vi "ManageScript.vi"(6 "Severity":string="Critical", 7 "ErrorIn Array":errorcluster[](array[cluster]), 10 "Script Locations":path[](array[path])) -> (0 "ErrorOut Array":errorcluster[](array[cluster]))   [LabVIEW 2018, in "Test.lvclass"]
uses:
  Test.lvclass
  <vilib>/Utility/config.llb/NI_LVConfig.lvlib
  <userlib>/NIST/NISTErrorLib/NISTErrorLib.lvlib
panel:
  in  "Script to Edit":string[](array[string])
  out "Script to View":string
  in  "btnRead":bool
  out "Numeric Control":i32
  out "Array 4":bool[](array[boolean])
  in  "Save As":bool
  in  "Save Button":bool
  in  "Script Names":string[](array[string])
  in  "Close Button":bool
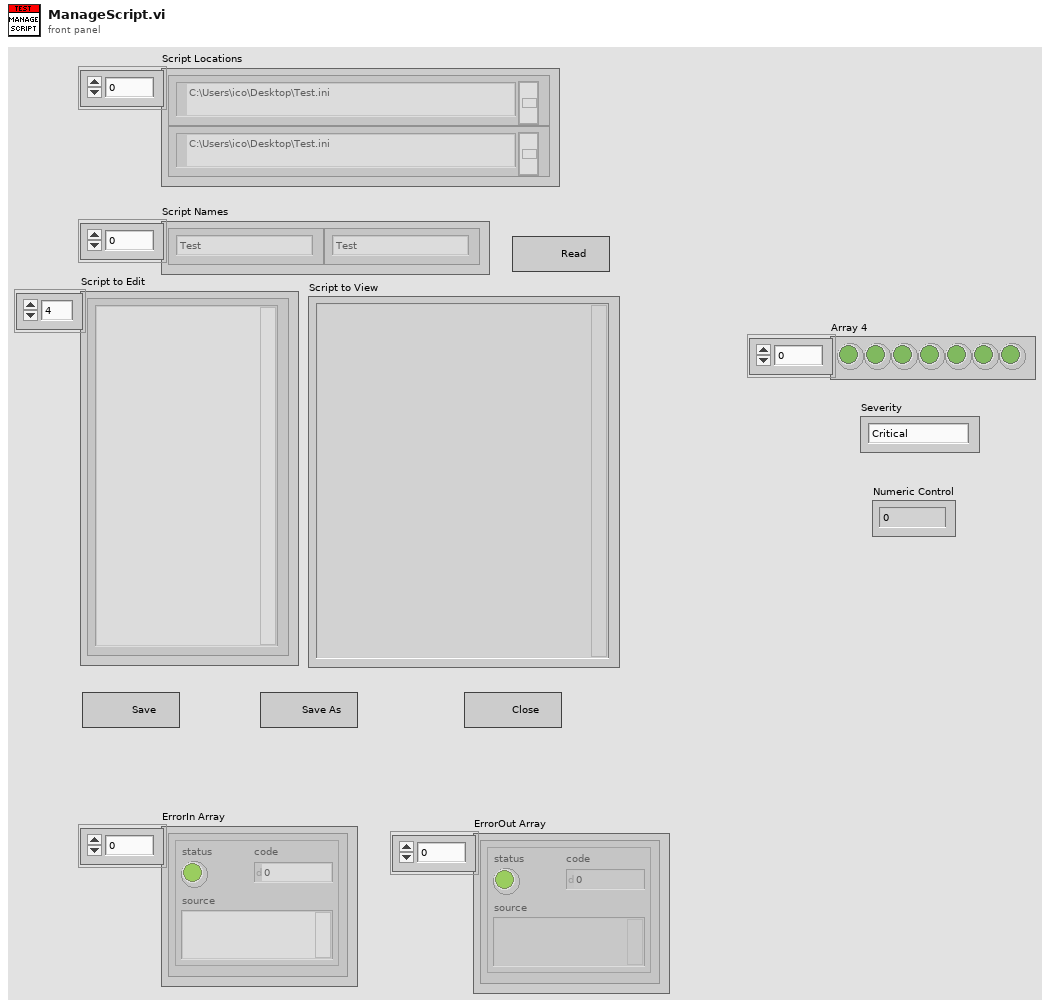
[diagram p1: front panel]
types:
  T1 = enum32{"Invalid", "Standard", "Closed", "Hidden", "Minimized", "Maximized"}
  T2 = enum32{"Invalid", "Default", "Floating", "Floating/Auto-Hide", "Modal"}
  T3 = typedef "NI_LVConfig.lvlib/Config Data RefNum.ctl" = refnum<k1>
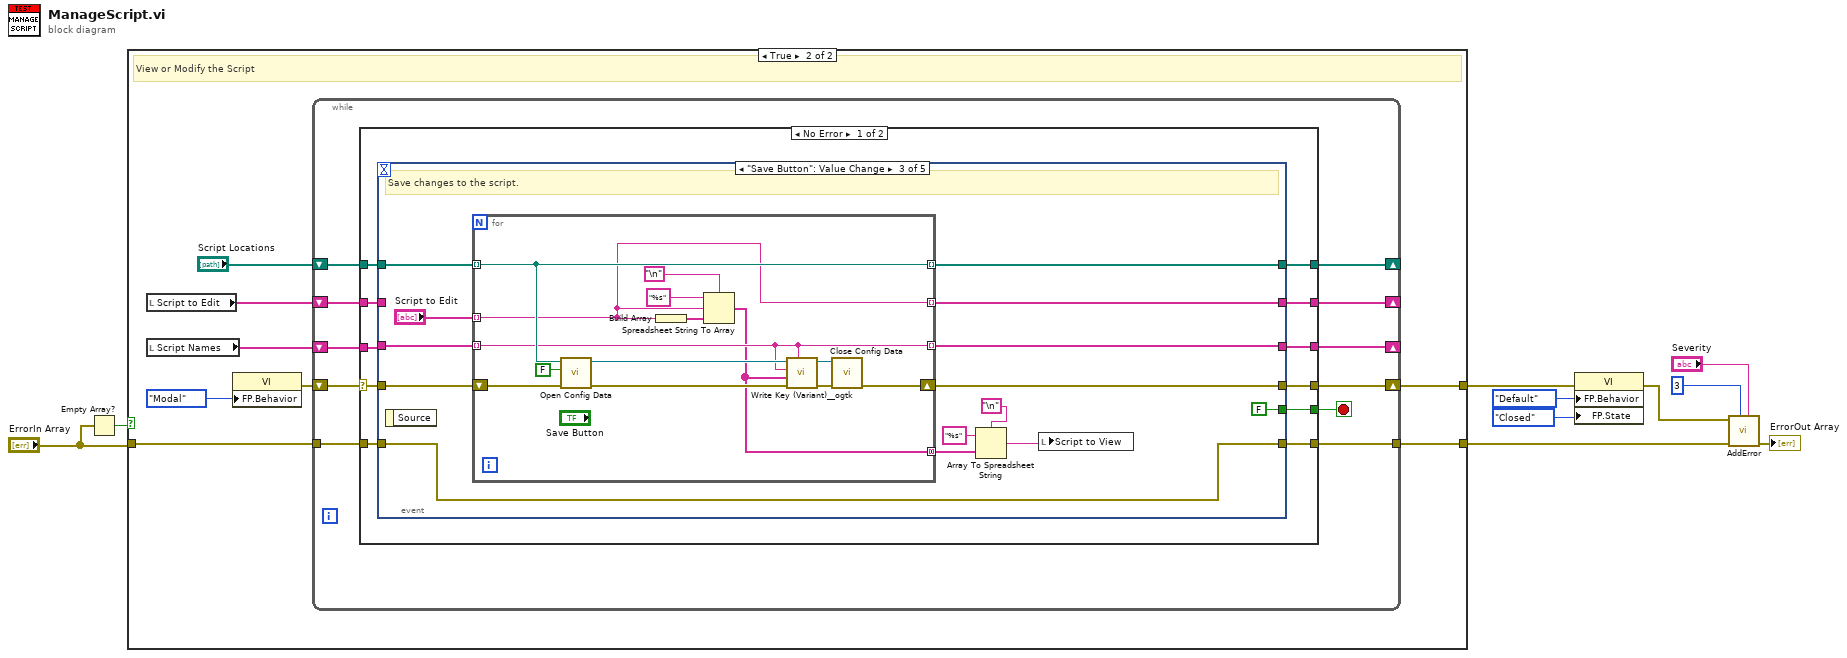
[diagram p0: block diagram]
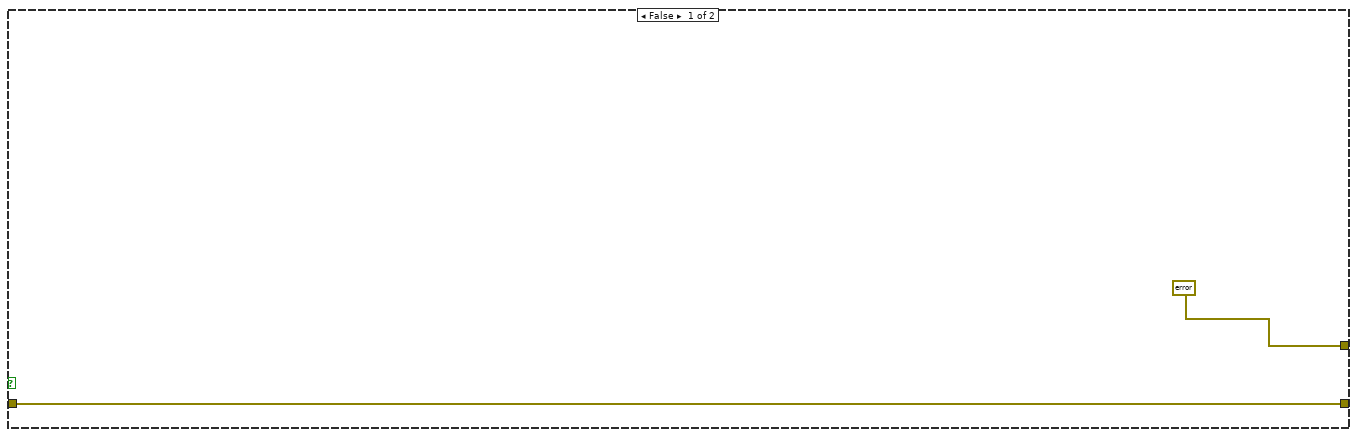
[diagram p2: hidden frame]
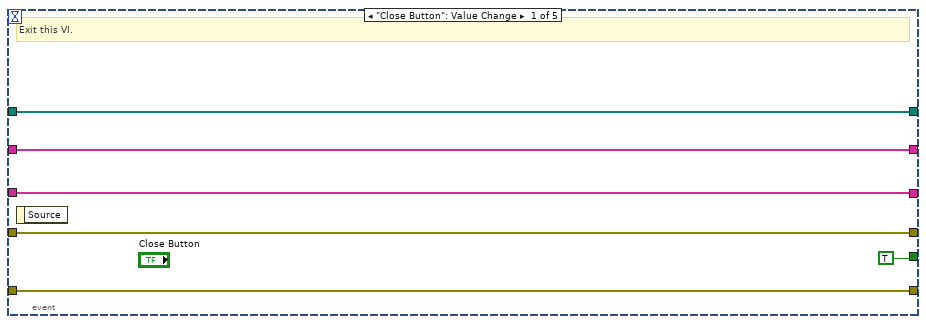
[diagram p3: hidden frame]
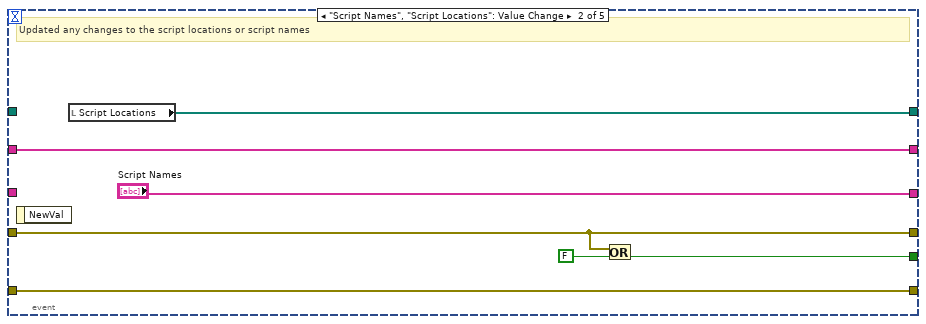
[diagram p4: hidden frame]
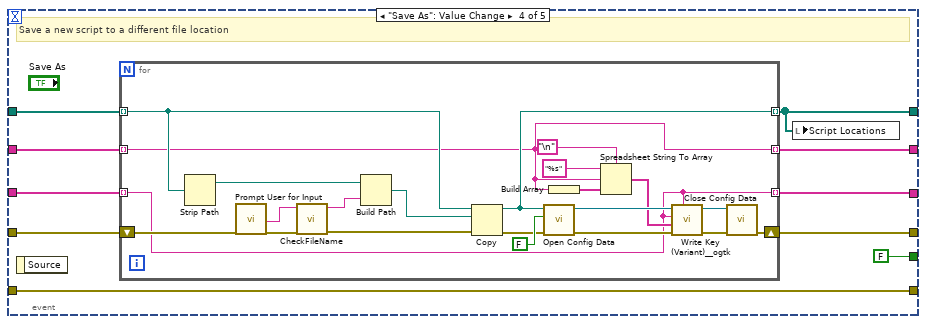
[diagram p5: hidden frame]
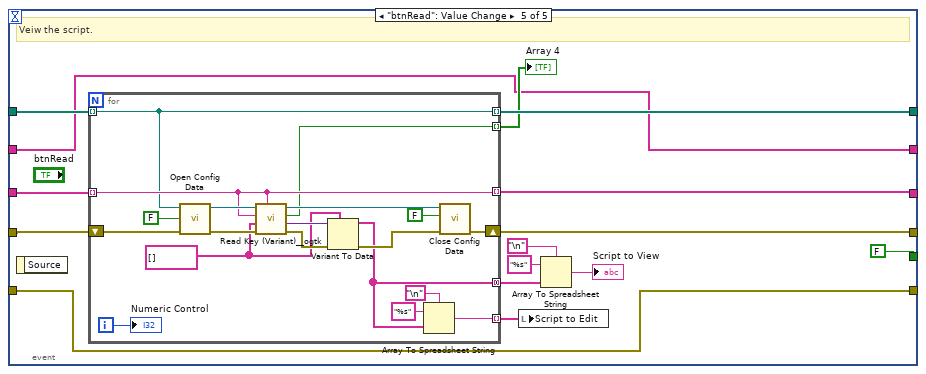
[diagram p6: hidden frame]
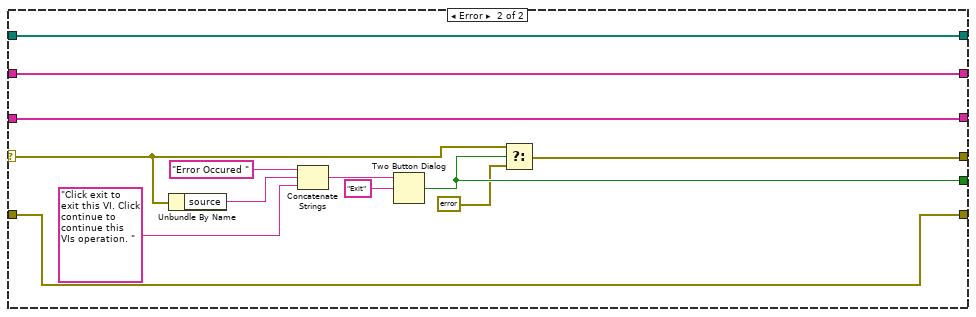
[diagram p7: hidden frame]
diagram:
  n1 = Empty Array?(array="ErrorIn Array") -> (empty?=w10:bool)
  n2 = case shown="True" w10 {
    tunnel: "ErrorIn Array" -> [w12 w20]
    tunnel: [w12 w14] -> w1
    tunnel: [errorcluster {"status"=FALSE, "code"=0, "source"=""} ("error out") w15] -> w3
    frame False {
    }
    frame True {
      # "View or Modify the Script"
      n3 = local read "Script to Edit"() -> (w16:string[])
      n4 = local read "Script Names"() -> (w17:string[])
      n5 = property class="VI"("FP.Behavior"=T2."Modal" ("Front Panel Window:Behavior")) -> (error out=w19:errorcluster)  [unwired: 2 in, 1 out]
      n6 = while {
        tunnel: w20 -> [w30]
        tunnel: [w29] -> w14
        shift-right: [w27] -> w15
        shift-left: w19 -> [w28]
        shift-right: [w25] -> _
        shift-left: "Script Locations" -> [w26]
        shift-right: [w23] -> _
        shift-left: w17 -> [w24]
        shift-right: [w21] -> _
        shift-left: w16 -> [w22]
        stop <- w31 stop-if-true
        n7 = case shown="No Error" w28 {
          selector: w28 -> [w39 w152]
          tunnel: [w42 w151] -> w31
          tunnel: w30 -> [w41 w156]
          tunnel: [w40 w156] -> w29
          tunnel: [w38 w153] -> w27
          tunnel: w26 -> [w37 w162]
          tunnel: [w36 w162] -> w25
          tunnel: w24 -> [w35 w160]
          tunnel: [w34 w160] -> w23
          tunnel: w22 -> [w33 w161]
          tunnel: [w32 w161] -> w21
          frame No Error {
            n8 = event shown="[2] \"Save Button\": Value Change" {
              selector: _ -> [_ _ _ _ _]
              dyn-events: _ -> [_ _ _ _ _]
              timeout: _ -> [_ _ _ _ _]
              tunnel: [TRUE w52 FALSE FALSE FALSE] -> w42
              tunnel: w41 -> [w48 w54 w60 w92 w126]
              tunnel: [w48 w54 w60 w92 w126] -> w40
              tunnel: w37 -> [w45 _ w68 w91 w128]
              tunnel: w35 -> [w44 _ w66 w90 w127]
              tunnel: w39 -> [w46 w51 w69 w93 w130]
              tunnel: [w46 w51 w64 w89 w129] -> w38
              tunnel: [w45 w49 w65 w84 w120] -> w36
              tunnel: [w44 "Script Names" w62 w87 w125] -> w34
              tunnel: w33 -> [w43 w50 _ w86 w117]
              tunnel: [w43 w50 w61 w85 w117] -> w32
              event "Close Button": Value Change {
                # "Exit this VI."
                n9 = event-data() -> ()  [unwired: 1 in, 1 out]
              }
              event "Script Names", "Script Locations": Value Change {
                # "Updated any changes to the script locations or script names"
                n10 = event-data() -> ()  [unwired: 1 in, 1 out]
                n11 = local read "Script Locations"() -> (w49:path[])
                n12 = Or(x=w51, y=FALSE) -> (x .or. y?=w52:bool)
              }
              event "Save Button": Value Change {
                # "Save changes to the script."
                n13 = event-data() -> ()  [unwired: 1 in, 1 out]
                n14 = for {
                  shift-right: [w77] -> w64
                  shift-left: w69 -> [w78]
                  tunnel: w68 -> [w73] mode=indexing
                  tunnel: "Script to Edit" -> [w71] mode=indexing
                  tunnel: w66 -> [w72] mode=indexing
                  tunnel: [w73] -> w65 mode=indexing
                  tunnel: [w72] -> w62 mode=indexing
                  tunnel: [w71] -> w61 mode=indexing
                  tunnel: [w70] -> w59 mode=concatenating
                  n15 = call <vilib>:"Open Config Data.vi"("error in (no error)"=w78, "create file if necessary (T)"=FALSE, "configuration file path"=w73) -> ("error out"=w82:errorcluster, "refnum"=w80:T3)  [unwired: 6 in, 1 out]
                  n16 = Build Array(w71) -> (w76:string[])
                  n17 = Spreadsheet String To Array(delimiter (Tab)="\n", format string="%s", spreadsheet string=w71, array type (2D Dbl)=w76) -> (array=w70:string[])
                  n18 = call <userlib>:"Write Key (Variant)__ogtk.vi"("section"=w72, "error in (no error)"=w82, "key-value"=w70, "key (optional)"=w72, "refnum"=w80) -> ("error out"=w81:errorcluster, "refnum out"=w79:T3)  [unwired: 5 in]
                  n19 = call <vilib>:"Close Config Data.vi"("error in (no error)"=w81, "refnum"=w79) -> ("error out"=w77:errorcluster)  [unwired: 8 in, 1 out]
                }
                n20 = Array To Spreadsheet String(delimiter (Tab)="\n", array=w59, 3:"%s" ("format string")) -> (spreadsheet string=w56:string)
                n21 = local write "Script to View"(w56) -> ()
              }
              event "Save As": Value Change {
                # "Save a new script to a different file location"
                n22 = event-data() -> ()  [unwired: 1 in, 1 out]
                n23 = for {
                  shift-right: [w110] -> w89
                  shift-left: w93 -> [w102]
                  tunnel: w91 -> [w101] mode=indexing
                  tunnel: w86 -> [w98] mode=indexing
                  tunnel: w90 -> [w99] mode=indexing
                  tunnel: [w100] -> w84 mode=indexing
                  tunnel: [w99] -> w87 mode=indexing
                  tunnel: [w98] -> w85 mode=indexing
                  n24 = Strip Path(path=w101) -> (stripped path=w104:path)  [unwired: 1 out]
                  n25 = call "Prompt User for Input"("error in (no error)"=w102) -> ("File Name"=w96:string, "error out"=w97:errorcluster)  [unwired: 16 in, 1 out]
                  n26 = call "CheckFileName.vi"("Error In"=w97, "File Name in"=w96) -> ("Error Out"=w94:errorcluster, "File Name out"=w95:string)  [unwired: 8 in]
                  n27 = Build Path(base path=w104, name or relative path=w95) -> (appended path=w105:path)
                  n28 = Copy(8:w94, 10:w105, 11:w101) -> (0:w103:errorcluster, 3:w100:path)  [unwired: 2 in, 1 out]
                  n29 = call <vilib>:"Open Config Data.vi"("error in (no error)"=w103, "create file if necessary (T)"=FALSE, "configuration file path"=w100) -> ("error out"=w114:errorcluster, "refnum"=w112:T3)  [unwired: 6 in, 1 out]
                  n30 = Build Array(w98) -> (w109:string[])
                  n31 = Spreadsheet String To Array(delimiter (Tab)="\n", format string="%s", spreadsheet string=w98, array type (2D Dbl)=w109) -> (array=w106:string[])
                  n32 = call <userlib>:"Write Key (Variant)__ogtk.vi"("section"=w99, "error in (no error)"=w114, "key-value"=w106, "key (optional)"=w99, "refnum"=w112) -> ("error out"=w113:errorcluster, "refnum out"=w111:T3)  [unwired: 5 in]
                  n33 = call <vilib>:"Close Config Data.vi"("error in (no error)"=w113, "refnum"=w111) -> ("error out"=w110:errorcluster)  [unwired: 8 in, 1 out]
                }
                n34 = local write "Script Locations"(w84) -> ()
              }
              event "btnRead": Value Change {
                # "Veiw the script."
                n35 = event-data() -> ()  [unwired: 1 in, 1 out]
                n36 = for {
                  tunnel: w128 -> [w138] mode=indexing
                  tunnel: w127 -> [w139] mode=indexing
                  shift-right: [w147] -> w129
                  shift-left: w130 -> [w148]
                  tunnel: [w139] -> w125 mode=indexing
                  tunnel: [w132] -> w121 mode=concatenating
                  tunnel: [w138] -> w120 mode=indexing
                  tunnel: [w135] -> w119 mode=indexing
                  tunnel: [w131] -> w116 mode=indexing
                  i -> [w136]
                  w137 = string[] []
                  n37 = call <vilib>:"Open Config Data.vi"("error in (no error)"=w148, "create file if necessary (T)"=FALSE, "configuration file path"=w138) -> ("error out"=w144:errorcluster, "refnum"=w142:T3)  [unwired: 6 in, 1 out]
                  n38 = call <userlib>:"Read Key (Variant)__ogtk.vi"("section"=w139, "error in (no error)"=w144, "type"=w137, "key (optional)"=w139, "refnum"=w142) -> ("error out"=w145:errorcluster, "key-value"=w146:variant, "found?"=w135:bool, "refnum out"=w141:T3)  [unwired: 3 in]
                  n39 = Variant To Data(error in=w145, type=w137, Variant=w146) -> (data=w132:string[], error out=w143:errorcluster)
                  n40 = Array To Spreadsheet String(delimiter (Tab)="\n", array=w132, 3:"%s" ("format string")) -> (spreadsheet string=w131:string)
                  n41 = call <vilib>:"Close Config Data.vi"("error in (no error)"=w143, "write file if changed (T)"=FALSE, "refnum"=w141) -> ("error out"=w147:errorcluster)  [unwired: 7 in, 1 out]
                  "Numeric Control" <- w136
                }
                "Array 4" <- w119
                n42 = local write "Script to Edit"(w116) -> ()
                n43 = Array To Spreadsheet String(delimiter (Tab)="\n", array=w121, 3:"%s" ("format string")) -> (spreadsheet string=→"Script to View":string)
              }
            }
          }
          frame Error {
            n44 = Unbundle By Name(w152) -> ("source"=w158:string)
            n45 = Concatenate Strings("Error Occured " ("message"), w158, "Click exit to exit this VI. Click  continue to continue this VIs operation. " ("message")) -> (w154:string)
            n46 = Two Button Dialog(message=w154, 2:"Exit" ("T button name (\"OK\")")) -> (T button?=w151:bool)  [unwired: 1 in]
            n47 = Select(t=w152, s=w151, f=errorcluster {"status"=FALSE, "code"=0, "source"=""}) -> (s? t:f=w153:errorcluster)
          }
        }
      }
    }
  }
  n48 = property class="VI"(error in=w3, "FP.Behavior"=T2."Default" ("Front Panel Window:Behavior"), "FP.State"=T1."Closed" ("Front Panel Window:State")) -> (error out=w8:errorcluster)  [unwired: 1 in, 1 out]
  n49 = call <userlib>:"AddError.vi"("Severity"="Severity", "Priority"=u8 3, "ErrorArray"=w1, "error in (no error)"=w8) -> ("ErrorArray"=→"ErrorOut Array":errorcluster[])  [unwired: 6 in, 1 out]
